vi "LC Control Set Value.vi"(8 "error in (no error)":errorcluster caption="Error In") -> (0 "error out":errorcluster caption="Error Out")   [LabVIEW 2020]
uses:
  LC Single Control Information.ctl
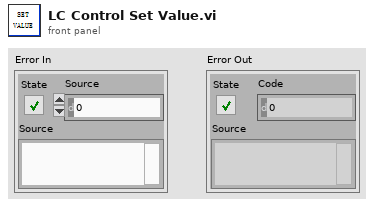
[diagram p1: front panel]
types:
  T1 = typedef "LC Single Control Information.ctl" = cluster{"VI Path":string, "VI Name":string, "Control Name":string, "Property Type":string, "Language":string, "Content":string}
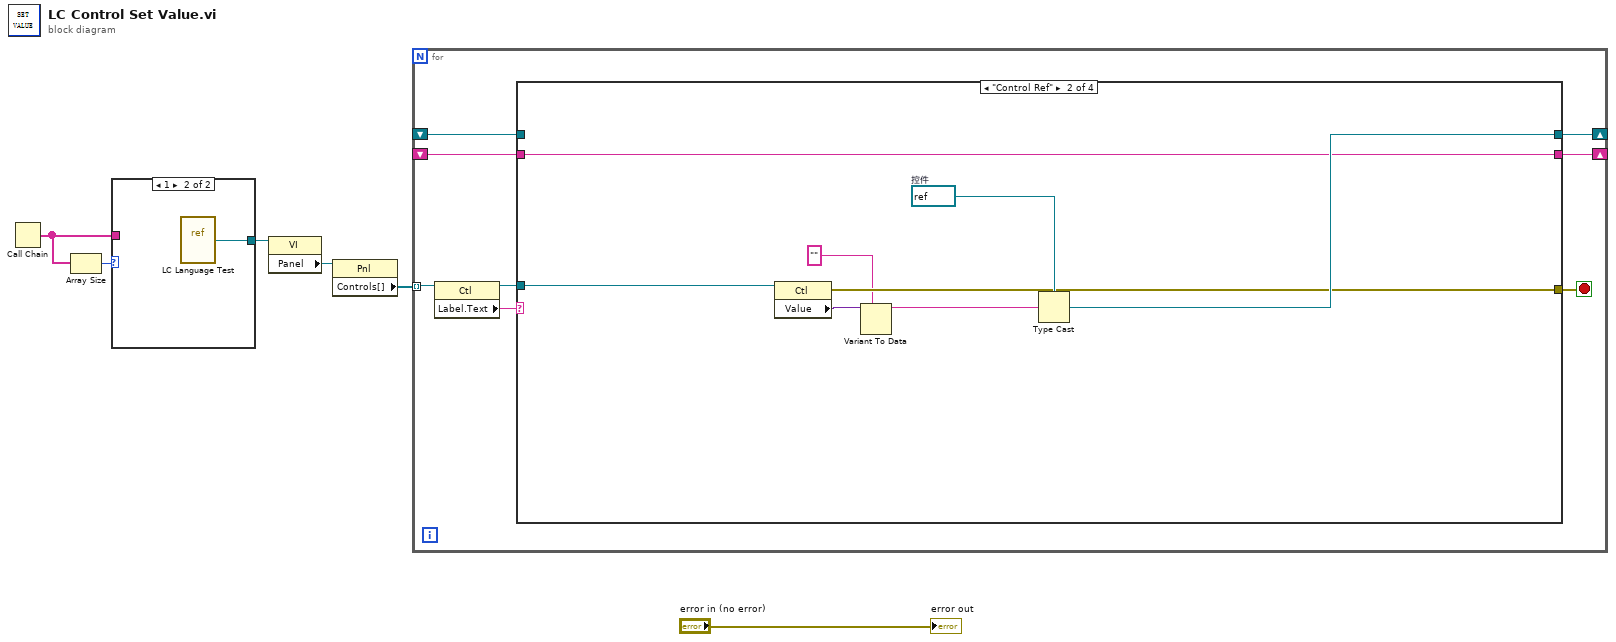
[diagram p0: block diagram]
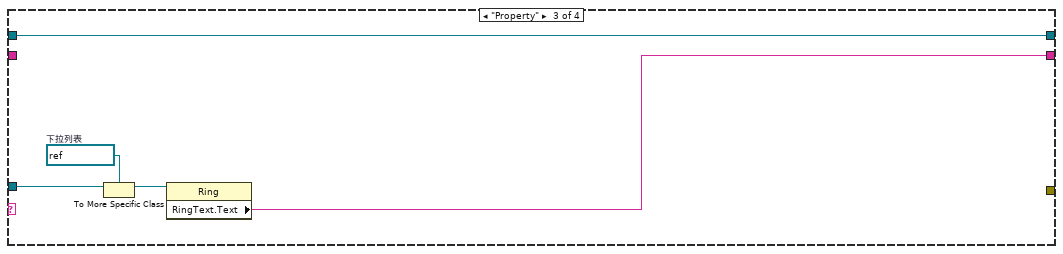
[diagram p3: hidden frame]
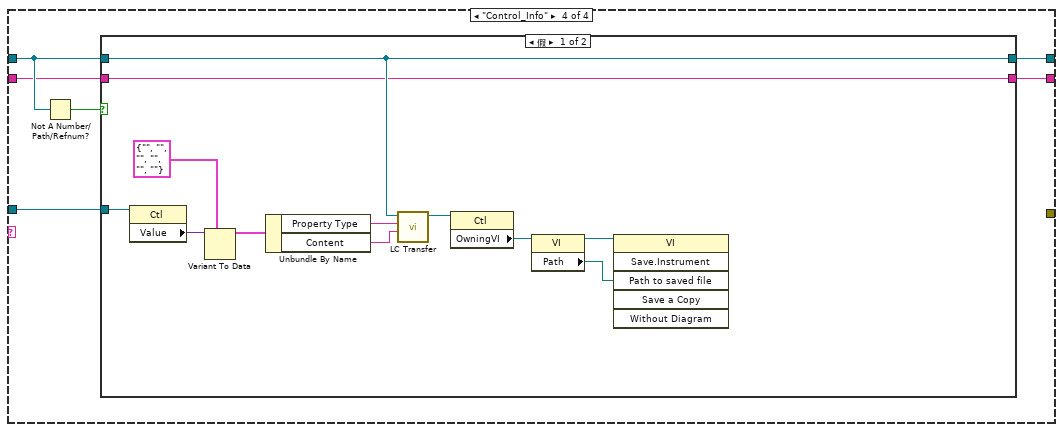
[diagram p4: hidden frame]
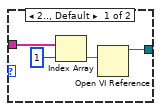
[diagram p6: hidden frame]
diagram:
  n1 = Call Chain() -> (call chain=w5:string[])
  n2 = Array Size(array=w5) -> (size(s)=w6:i32)
  n3 = case shown="1" w6 {
    tunnel: [w8 w11] -> w3
    tunnel: w5 -> [w7 _]
    frame 2.., Default {
      n4 = Index Array(array=w7, index=1 ("索引")) -> (element=w9:string)
      n5 = Open VI Reference(vi path=w9) -> (vi reference=w8:refnum<vi>)  [unwired: 5 in, 1 out]
    }
    frame 1 {
      n6 = vi-ref "LC Language Test.vi"() -> (w11:refnum<vi>)
    }
  }
  n7 = property class="VI"(reference=w3) -> ("Panel"=w4:refnum<vi>)  [unwired: 1 in, 2 out]
  n8 = property class="Pnl"(reference=w4) -> ("Controls[]"=w2:refnum<vi>[])  [unwired: 1 in, 2 out]
  n9 = for {
    tunnel: w2 -> [w19] mode=indexing
    shift-right: [w16] -> _
    shift-left: _ -> [w15]
    shift-right: [w13] -> _
    shift-left: _ -> [w12]
    stop <- w14 stop-if-true
    n10 = property class="Ctl"(reference=w19) -> (reference out=w17:refnum<vi>, "Label.Text"=w18:string)  [unwired: 1 in, 1 out]
    n11 = case shown="\"Control Ref\"" w18 {
      tunnel: w17 -> [_ w25 w33 w40]
      tunnel: [w21 w28 w34 w37] -> w16
      tunnel: w15 -> [w21 _ w34 w39]
      tunnel: [_ w27 _ _] -> w14
      tunnel: [w20 w26 w30 w35] -> w13
      tunnel: w12 -> [w20 w26 _ w36]
      frame "eee", Default {
      }
      frame "Control Ref" {
        w29 = refnum<vi> refnum  # 控件
        n12 = property class="Ctl"(reference=w25) -> (error out=w27:errorcluster, "Value"=w24:variant)  [unwired: 1 in, 1 out]
        n13 = Variant To Data(type="", Variant=w24) -> (data=w22:string)  [unwired: 1 in, 1 out]
        n14 = Type Cast(type=w29, x=w22) -> (*(type *) &x=w28:refnum<vi>)
      }
      frame "Property" {
        w32 = refnum<vi> refnum  # 下拉列表
        n15 = To More Specific Class(target class=w32, reference=w33) -> (specific class reference=w31:refnum<vi>)  [unwired: 1 in, 1 out]
        n16 = property class="Ring"(reference=w31) -> ("RingText.Text"=w30:string)  [unwired: 1 in, 2 out]
      }
      frame "Control_Info" {
        n17 = Not A Number/Path/Refnum?(number/path/refnum=w39) -> (NaN/Path/Refnum?=w38:bool)
        n18 = case shown="假" w38 {
          tunnel: w40 -> [w52 _]
          tunnel: w39 -> [w50 w54]
          tunnel: [w50 w54] -> w37
          tunnel: w36 -> [w49 w53]
          tunnel: [w49 w53] -> w35
          frame False {
            n19 = property class="Ctl"(reference=w52) -> ("Value"=w51:variant)  [unwired: 1 in, 2 out]
            n20 = Variant To Data(type=T1 {"VI Path"="", "VI Name"="", "Control Name"="", "Property Type"="", "Language"="", "Content"=""} ("Control_Info"), Variant=w51) -> (data=w48:T1)  [unwired: 1 in, 1 out]
            n21 = Unbundle By Name(w48) -> ("Property Type"=w42:string, "Content"=w43:string)
            n22 = call "LC Transfer.vi"("Value In"=w43, "Property"=w42, "Ctl Ref In"=w50) -> ("Ctl Ref Out"=w41:refnum<vi>)  [unwired: 6 in, 2 out]
            n23 = property class="Ctl"(reference=w41) -> ("OwningVI"=w46:refnum<vi>)  [unwired: 1 in, 2 out]
            n24 = property class="VI"(reference=w46) -> (reference out=w45:refnum<vi>, "Path"=w44:path)  [unwired: 1 in, 1 out]
            n25 = invoke class="VI" method="Save.Instrument"(reference=w45, "Path to saved file"=w44) -> ()  [unwired: 4 in, 6 out]
          }
          frame True {
          }
        }
      }
    }
  }
  "error out" <- "error in (no error)"
